vi "DataLog-Initialize.vi"(0 "Folder":path, 5 "Name":string, 7 "Cols":i32, 9 "Length":i32=10000, 11 "insert date":bool=TRUE) -> (4 "state":T1, 15 "error out":errorcluster)   [LabVIEW 2020]
uses:
  DataLog-State.ctl
  <vilib>/Utility/sysdir.llb/System Directory Type.ctl
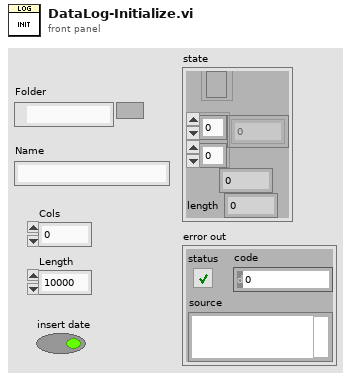
[diagram p1: front panel]
types:
  T1 = typedef "DataLog-State.ctl" = cluster{"file":refnum<file>, "data":dbl[][], "index":i32, "length":i32}
  T2 = enum16{"open", "replace", "create", "open or create", "replace or create", "replace or create with confirmation"}
  T3 = typedef "System Directory Type.ctl" = i32
  T4 = cluster{"refnum out":refnum<file>, dbl[][], i32, "Length":i32}
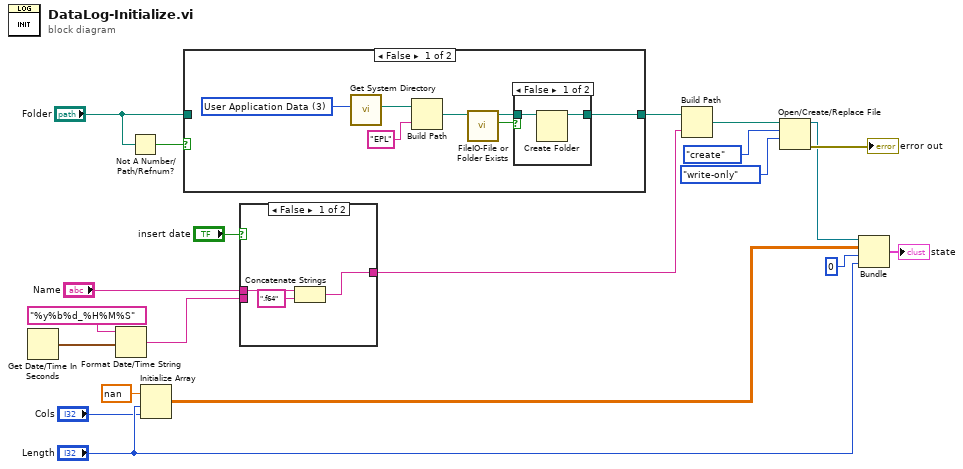
[diagram p0: block diagram]
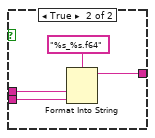
[diagram p2: hidden frame]
diagram:
  n1 = Get Date/Time In Seconds() -> (seconds since 1Jan1904=w17:timestamp)
  n2 = Format Date/Time String(time format string (%c)="%y%b%d_%H%M%S", seconds (now)=w17) -> (date/time string=w15:string)  [unwired: 1 in]
  n3 = Not A Number/Path/Refnum?(number/path/refnum="Folder") -> (NaN/Path/Refnum?=w20:bool)
  n4 = Initialize Array(nan ("element"), "Length", "Cols") -> (w6:dbl[][])
  n5 = case shown="False" w20 {
    tunnel: [w21 w31] -> w14
    tunnel: "Folder" -> [_ w31]
    frame False {
      w22 = T3 3 items=["User Home", "User Desktop", "User Documents", "User Application Data", "User Preferences", "User Temporary", "Public Documents", "Public Application Data", "Public Preferences", "System Core Libraries", "System Installed Libraries", "Application Files", "Boot Volume Root"] ("system directory type")
      n6 = call <vilib>:"Get System Directory.vi"("system directory type"=w22) -> ("system directory"=w23:path)  [unwired: 10 in]
      n7 = Build Path(base path=w23, name or relative path="EPL") -> (appended path=w25:path)
      n8 = call "FileIO-File or Folder Exists.vi"("path"=w25) -> ("Directory?"=w26:bool, "dup path"=w27:path)  [unwired: 7 in, 2 out]
      n9 = case shown="False" w26 {
        tunnel: w27 -> [w29 w30]
        tunnel: [w28 w30] -> w21
        frame False {
          n10 = Create Folder(path (use dialog)=w29) -> (created path=w28:path)  [unwired: 2 in, 2 out]
        }
        frame True {
        }
      }
    }
    frame True {
    }
  }
  n11 = case shown="False" "insert date" {
    tunnel: "Name" -> [w34 w37]
    tunnel: w15 -> [_ w36]
    tunnel: [w33 w35] -> w13
    frame False {
      n12 = Concatenate Strings(w34, ".f64" ("string")) -> (w33:string)
    }
    frame True {
      n13 = Format Into String(format string="%s_%s.f64", w37, w36) -> (resulting string=w35:string)  [unwired: 2 in, 1 out]
    }
  }
  n14 = Build Path(base path=w14, name or relative path=w13) -> (appended path=w12:path)
  n15 = Open/Create/Replace File(file path (use dialog)=w12, operation (0:open)=T2."create", access (0:read/write)=enum16{"read/write", "read-only", "write-only"}."write-only") -> (refnum out=w8:refnum<file>, error out=→"error out":errorcluster)  [unwired: 3 in, 1 out]
  n16 = Bundle("refnum out"=w8, w6, 0, "Length"="Length") -> (→"state":T4)  [unwired: 1 in]
